vi "FROMBASETOBALLRACK.vi"   [LabVIEW 2016, in "Test2.lvrbt"]
uses:
  Test2.lvrbt
  <vilib>/NXT/Hardware/Plugins/Tetrix DC Motor/TetrixDCMotorAddress.ctl
  <vilib>/NXT/Hardware/Plugins/Tetrix 180 deg Servo/Tetrix180ServoAddress.ctl
  <vilib>/NXT/NXTIO Xnodes/NXTIONodeSubVIs/TETRIX IO Move Servos.vi
  <vilib>/NXT/Dual Mode Library/Waits/Wait_Num.vi
  <vilib>/NXT/NXTIO Xnodes/NXTIONodeSubVIs/TETRIX IO Move DC Motors.vi
  <vilib>/NXT/NXTIO Xnodes/NXTIONodeSubVIs/TETRIX IO Stop DC Motors.vi
  <vilib>/NXT/NXTIO Xnodes/AddressXNode/NXTIOAddress.xnode
  <vilib>/NXT/Subs/LVHSConnector.ctl
  <vilib>/NXT/NXTIO Xnodes/NXTIOXNode/NXTIO.xnode
  <vilib>/NXT/LegoClasses/BrickReference/BrickReference.lvclass
types:
  T1 = typedef "Tetrix180ServoAddress.ctl" = i32
  T2 = cluster{"Tetrix180Servo":T1, "Tetrix180Servo":T1, "Tetrix180Servo":T1, "Tetrix180Servo":T1, "Tetrix180Servo":T1, "Tetrix180Servo":T1}
  T3 = typedef "LVHSConnector.ctl" = refnum<class "BrickReference.lvclass">
  T4 = typedef "TetrixDCMotorAddress.ctl" = i32
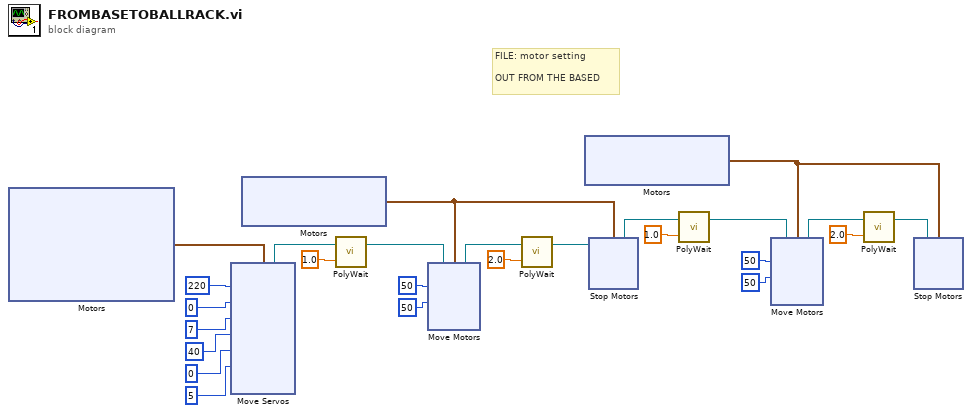
[diagram p0: block diagram]
diagram:
  # "FILE: motor setting\n\nOUT FROM THE BASED"
  n1 = xnode "Motors"() -> ("Motor"=w11:T2)
  n2 = xnode "Move Servos"("Position 6"=u8 5, "Position 5"=u8 0, "Position 4"=u8 40, "Position 3"=u8 7, "Position 2"=u8 0, "Position 1"=u8 220, "Motors"=w11) -> ("NXT/EV3"=w9:T3)  [unwired: 1 in]
  n3 = xnode "Motors"() -> ("Motor"=w15:cluster{"TetrixDCMotor":T4, "TetrixDCMotor":T4})
  n4 = call-poly <vilib>:"PolyWait.vi"("Time (1 sec)"=sgl 1.0, "NXT/EV3"=w9) -> ("NXT/EV3"=w8:T3)  [unwired: 2 in]
  n5 = xnode "Move Motors"("Power/Speed 2"=i8 50, "Power/Speed 1"=i8 50, "Motors"=w15, "NXT/EV3"=w8) -> ("NXT/EV3"=w18:T3)
  n6 = call-poly <vilib>:"PolyWait.vi"("Time (1 sec)"=sgl 2.0, "NXT/EV3"=w18) -> ("NXT/EV3"=w16:T3)  [unwired: 2 in]
  n7 = xnode "Motors"() -> ("Motor"=w1:cluster{"TetrixDCMotor":T4, "TetrixDCMotor":T4})
  n8 = xnode "Stop Motors"("Motors"=w15, "NXT/EV3"=w16) -> ("NXT/EV3"=w14:T3)
  n9 = call-poly <vilib>:"PolyWait.vi"("Time (1 sec)"=sgl 1.0, "NXT/EV3"=w14) -> ("NXT/EV3"=w12:T3)  [unwired: 2 in]
  n10 = xnode "Move Motors"("Power/Speed 2"=i8 50, "Power/Speed 1"=i8 50, "Motors"=w1, "NXT/EV3"=w12) -> ("NXT/EV3"=w23:T3)
  n11 = call-poly <vilib>:"PolyWait.vi"("Time (1 sec)"=sgl 2.0, "NXT/EV3"=w23) -> ("NXT/EV3"=w21:T3)  [unwired: 2 in]
  n12 = xnode "Stop Motors"("Motors"=w1, "NXT/EV3"=w21) -> ()  [unwired: 1 out]
